vi "Create Spawn.vi"(10 "DVR":refnum<data-value>) -> (3 "Class Out":refnum<class "Spawn.lvclass">)   [LabVIEW 2020, in "Spawn.lvclass"]
uses:
  Spawn/Spawn.lvclass
  C:/dev/IlluminatedG/sol-squarebattle/Squares/Robert Mortensen/Crosswinds/Crosswinds.lvclass
  DVR Cluster.ctl
  Spot Cluster.ctl
  State Enum.ctl
  Role Enum.ctl
  Type Defs/Direction Enum.ctl
  Crosswinds.lvclass/Crosswinds.ctl
  Spawn/Spawn.lvclass/Spawn.ctl
  Write DVR.vi
  Crosswinds.lvclass
  Type Defs/SB Type Defs.lvlib
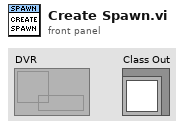
[diagram p1: front panel]
types:
  T1 = typedef "Crosswinds.lvclass/DVR Cluster.ctl" = cluster{"Map":T2[][], "Roles":T4[][], "RD":T5, "Buffer":i32, "Pattern":i32, "Spawn Points":cluster{"Row":i32, "Column":i32}[], "Start Row":i32, "Start Column":i32}
  T2 = typedef "Crosswinds.lvclass/Spot Cluster.ctl" = cluster{"State":T3, "Round":i32}
  T3 = typedef "Crosswinds.lvclass/State Enum.ctl" = enum16{"Attacked", "Occupied", "Fresh Grave", "Empty Child", "Empty Move", "Unexplored", "Empty Parent", "Grave", "Enemy"}
  T4 = typedef "Crosswinds.lvclass/Role Enum.ctl" = enum16{"P", "C", "M"}
  T5 = typedef "SB Type Defs.lvlib/Direction Enum.ctl" = enum16{"NW", "N", "NE", "E", "SE", "S", "SW", "W"}
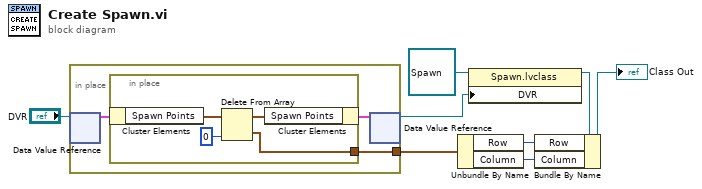
[diagram p0: block diagram]
diagram:
  n1 = in-place {
    in-place-border: [w9] -> w8
    n2 = in-place-dvr #1("DVR") -> (w11:T1)  [unwired: 1 out]
    n3 = in-place {
      in-place-border: [w12] -> w9
      n4 = in-place-cluster #2(w11) -> ("Spawn Points"=w15:cluster{"Row":i32, "Column":i32}[])
      n5 = Delete From Array(array=w15, index=0) -> (deleted portion=w12:cluster{"Row":i32, "Column":i32}, array with subset deleted=w14:cluster{"Row":i32, "Column":i32}[])  [unwired: 1 in]
      n6 = in-place-cluster #2("Spawn Points"=w14) -> (w10:T1)
    }
    n7 = in-place-dvr #1(w10) -> (w1:refnum<data-value>)  [unwired: 1 out]
  }
  n8 = Unbundle By Name(w8) -> ("Row"=w5:i32, "Column"=w4:i32)
  n9 = property class="Spawn.lvclass"(reference=refnum<class "Spawn.lvclass"> refnum ("Spawn.lvclass"), "DVR"=w1) -> (reference out=w2:refnum<class "Spawn.lvclass">)  [unwired: 1 in, 1 out]
  n10 = Bundle By Name(cluster=w2, "Row"=w5, "Column"=w4) -> (→"Class Out":refnum<class "Spawn.lvclass">)
